vi "correctDelays.vi"(8 "error in (no error)":errorcluster, 10 "eventStringArray in":string[][](array[string]), 11 "ScriptEventList in":refnum<class "ScriptEventList.lvclass">) -> (0 "error out":errorcluster, 2 "eventStringArray":string[][](array[string]), 3 "ScriptEventList out":refnum<class "ScriptEventList.lvclass">)   [LabVIEW 2011, in "Tools.lvlib" / "Scripting.lvlib" / "ScriptEventList.lvclass"]
uses:
  ScriptEventList.lvclass
  ScriptEventList.lvclass/ScriptEventList.ctl
  ScriptEvent.lvclass
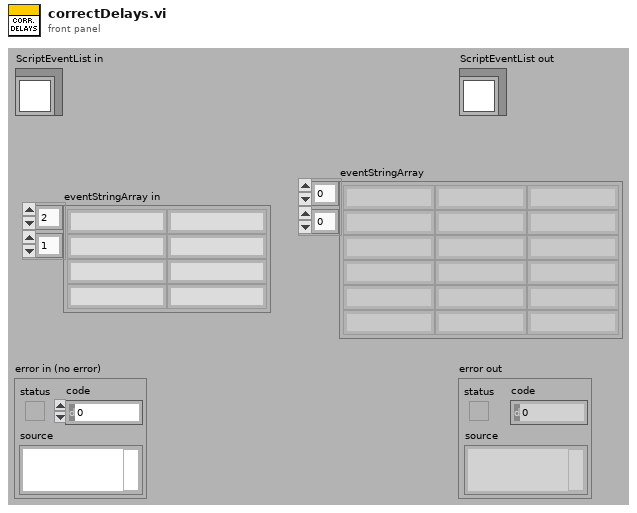
[diagram p1: front panel]
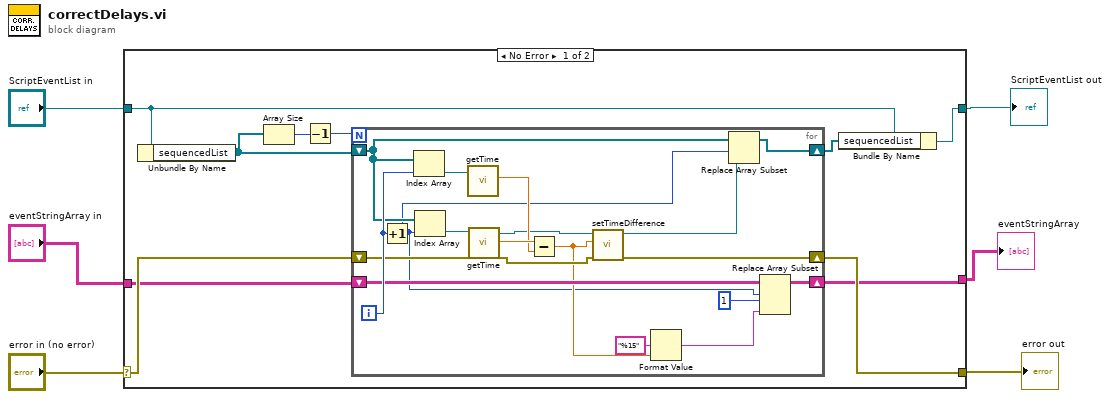
[diagram p0: block diagram]
diagram:
  n1 = case shown="No Error" "error in (no error)" {
    selector: "error in (no error)" -> [w13 w37]
    tunnel: [w12 w37] -> w5
    tunnel: [w10 w36] -> w3
    tunnel: "ScriptEventList in" -> [w11 w36]
    tunnel: "eventStringArray in" -> [w8 _]
    tunnel: [w7 _] -> w1
    frame No Error {
      n2 = Unbundle By Name(w11) -> ("sequencedList"=w14:refnum<class "ScriptEvent.lvclass">[])
      n3 = Array Size(array=w14) -> (size(s)=w16:i32)
      n4 = Decrement(x=w16) -> (x-1=w15:i32)
      n5 = for {
        N: w15 -> [_]
        shift-right: [w24] -> w9
        shift-left: w14 -> [w28]
        shift-right: [w26] -> w12
        shift-left: w13 -> [w25]
        shift-right: [w19] -> w7
        shift-left: w8 -> [w23]
        i -> [w35]
        n6 = Increment(x=w35) -> (x+1=w17:i32)
        n7 = Index Array(array=w28, index=w35) -> (element=w34:refnum<class "ScriptEvent.lvclass">)
        n8 = Index Array(array=w28, index=w17) -> (element=w33:refnum<class "ScriptEvent.lvclass">)
        n9 = call "getTime.vi"("ScriptEvent.lvclass in"=w34) -> ("time"=w31:dbl)  [unwired: 8 in, 2 out]
        n10 = call "getTime.vi"("error in (no error)"=w25, "ScriptEvent.lvclass in"=w33) -> ("error out"=w29:errorcluster, "time"=w32:dbl, "ScriptEvent.lvclass out"=w30:refnum<class "ScriptEvent.lvclass">)  [unwired: 7 in]
        n11 = Subtract(x=w32, y=w31) -> (x-y=w22:dbl)
        n12 = call "setTimeDifference.vi"("error in (no error)"=w29, "time difference"=w22, "ScriptEvent.lvclass in"=w30) -> ("error out"=w26:errorcluster, "ScriptEvent.lvclass out"=w27:refnum<class "ScriptEvent.lvclass">)  [unwired: 7 in]
        n13 = Format Value(format string="%15", value (0)=w22) -> (output string=w20:string)  [unwired: 1 in]
        n14 = Replace Array Subset(array=w28, new element=w27, index=w17) -> (w24:refnum<class "ScriptEvent.lvclass">[])
        n15 = Replace Array Subset(array=w23, new element=w20, index (row)=w17, index (col)=1) -> (w19:string[][])
      }
      n16 = Bundle By Name(cluster=w11, "sequencedList"=w9) -> (w10:refnum<class "ScriptEventList.lvclass">)
    }
    frame Error {
    }
  }
  "error out" <- w5
  "ScriptEventList out" <- w3
  "eventStringArray" <- w1
